vi "Memory.Pointer.Copy.vi"   [LabVIEW 2016, in "Memory Manager.lvlib" / "Memory.Pointer.lvclass"]
doc: "Copies <b>bytes to copy</b> of data from the memory address specified by <b>src pointer</b> to the memory address specified by <b>dst pointer</b>."
uses:
  Memory.Pointer.lvclass
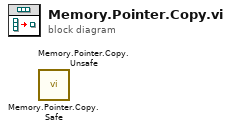
[diagram p0: block diagram]
diagram:
  n1 = call "Memory.Pointer.Copy.Safe.vi"() -> ()  [unwired: 8 in, 4 out]
  n2 = call "Memory.Pointer.Copy.Unsafe.vi"() -> ()  [unwired: 8 in, 4 out]
